vi "Clear.vi"(8 "error in (no error)":errorcluster, 11 "Digital Serial in":refnum<class "Digital Serial.lvclass">) -> (0 "error out":errorcluster)   [LabVIEW 2023, in "Digital Serial.lvclass"]
uses:
  Digital Serial.lvclass
  Digital Serial.lvclass/Digital Serial.ctl
  <vilib>/PDM Acquisition Toolkit/host/API/PDM Acquisition Toolkit.lvlib
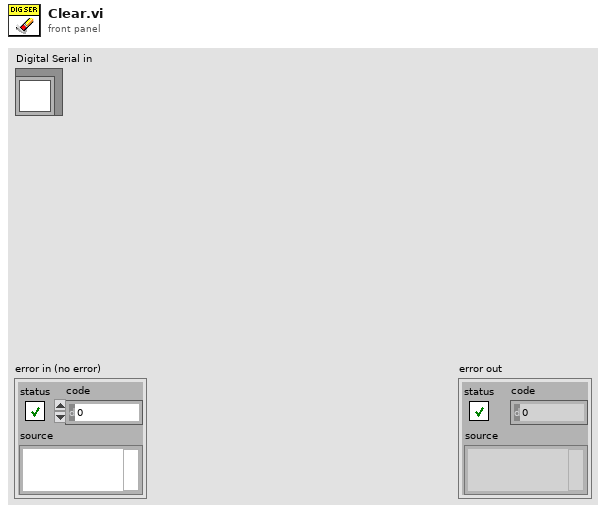
[diagram p1: front panel]
types:
  T1 = typedef "PDM Acquisition Class Library.lvlib/PCM Output Task.lvclass/PCM Output Task DVR.ctl" = refnum<data-value>
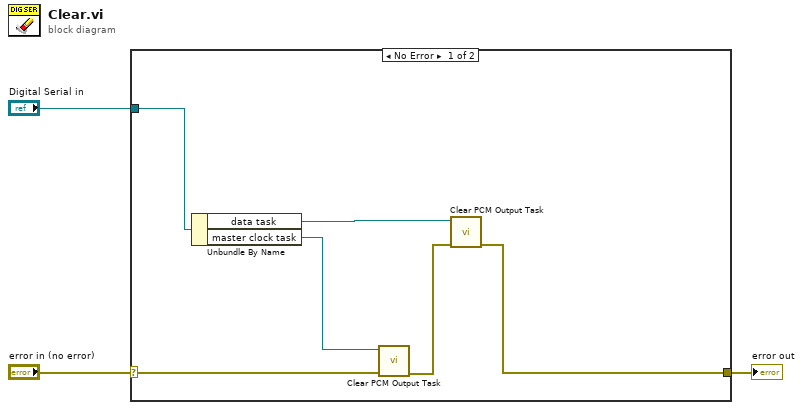
[diagram p0: block diagram]
diagram:
  n1 = case shown="No Error" "error in (no error)" {
    selector: "error in (no error)" -> [w8 w10]
    tunnel: [w7 w10] -> w2
    tunnel: "Digital Serial in" -> [w6 _]
    frame No Error {
      n2 = Unbundle By Name(w6) -> ("data task"=w5:T1, "master clock task"=w4:T1)
      n3 = call <vilib>:"Clear PCM Output Task.vi"("error in"=w8, "PCM output task in"=w4) -> ("error out"=w9:errorcluster)  [unwired: 9 in]
      n4 = call <vilib>:"Clear PCM Output Task.vi"("error in"=w9, "PCM output task in"=w5) -> ("error out"=w7:errorcluster)  [unwired: 9 in]
    }
    frame Error {
    }
  }
  "error out" <- w2
